vi "StressControl Data.vi"() -> (0 "Stress Control Data":T1={"Configuration"={"Stress Control VISA Session"="StrainMotor", "Axis"=0, "Motion"=0, "Destination (°)"=0.0, "Speed (°/s)"=4.0, "Position (°)"=25.0}, "Refnums"={"Instrument Status"=refnum, "Position"=refnum, "Mecahnism Motion"=refnum, "Destination"=refnum, "Apply Stress"=refnum, "Stop"=refnum, "Stress Control VISA"=refnum}, "Initialization"={"Update Visa Session"=FALSE, "Update Configuration"=FALSE, "Update Refnums"=FALSE, "Get Position"=FALSE}} {"Configuration"."Axis" min=1 max=3; "Configuration"."Position (°)" format="%.6g"; "Configuration"."Speed (°/s)" min=0.0 max=4.0 format="%.6f"; "Configuration"."Destination (°)" min=-2000000000.0 max=2000000000.0 format="%.6f"; "Configuration"."Motion" items=["Absolute", "Relative"]})   [LabVIEW 2014]
uses:
  StressControl Data.ctl
  StressControl Config.ctl
  StressControl Refnums.ctl
  StressControl Initialization.ctl
panel:
  # "LICENSED MATERIALS – PROPERTY OF IBM\nCopyright IBM Corp. 2016,\nALL RIGHTS RESERVED"
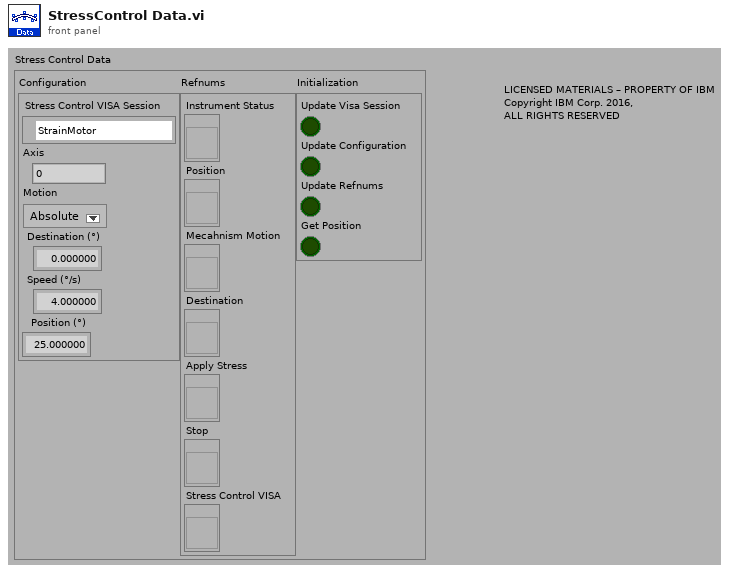
[diagram p1: front panel]
types:
  T1 = typedef "StressControl Data.ctl" = cluster{"Configuration":T2, "Refnums":T3, "Initialization":T4}
  T2 = typedef "StressControl Config.ctl" = cluster{"Stress Control VISA Session":refnum<visa-resource-name>, "Axis":i32, "Motion":u16, "Destination (°)":dbl, "Speed (°/s)":dbl, "Position (°)":dbl}
  T3 = typedef "StressControl Refnums.ctl" = cluster{"Instrument Status":refnum<vi>, "Position":refnum<vi>, "Mecahnism Motion":refnum<vi>, "Destination":refnum<vi>, "Apply Stress":refnum<vi>, "Stop":refnum<vi>, "Stress Control VISA":refnum<vi>}
  T4 = typedef "StressControl Initialization.ctl" = cluster{"Update Visa Session":bool, "Update Configuration":bool, "Update Refnums":bool, "Get Position":bool}
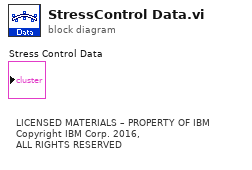
[diagram p0: block diagram]
diagram:
  # "LICENSED MATERIALS – PROPERTY OF IBM\nCopyright IBM Corp. 2016,\nALL RIGHTS RESERVED"
